vi "LogSpectra.vi"(7 "Area":i32, 8 "error in (no error)":errorcluster, 9 "50mA Spectra":cluster{"Wavelength":dbl[], "EL Spectrum":dbl[]}, 10 "20mA Spectra":cluster{"Wavelength":dbl[], "EL Spectrum":dbl[]}, 11 "LotData in":refnum<class "LotData.lvclass">) -> (0 "error out":errorcluster, 2 "Boolean":bool=TRUE, 3 "LotData out":refnum<class "LotData.lvclass">)   [LabVIEW 2012, in "LotData.lvclass"]
uses:
  LotData.lvclass
  <vilib>/addons/database/NI_Database_API.lvlib
  <vilib>/addons/database/Connection.llb/DB Tools Open Connec (Path).vi
  <vilib>/addons/database/Auxilliary.llb/DB Tools Parameter Dir.ctl
  <vilib>/addons/database/Auxilliary.llb/DB Tools DataTypes.ctl
  <vilib>/addons/database/Auxilliary.llb/DB Tools Parameter Info.ctl
  <vilib>/addons/database/Command.llb/Cmd Set Parameter Value (C).vi
  <vilib>/addons/database/Command.llb/Cmd Delete.vi
  <vilib>/LVH/i3 JSON/i3-json.lvlib
  <vilib>/LVH/i3 JSON/JSON Generation/Create Value Files/Create Value - 1D Array Double.vi
  <vilib>/addons/database/Command.llb/Cmd Execute.vi
  <vilib>/addons/database/Recordset.llb/Rec Destroy - Command.vi
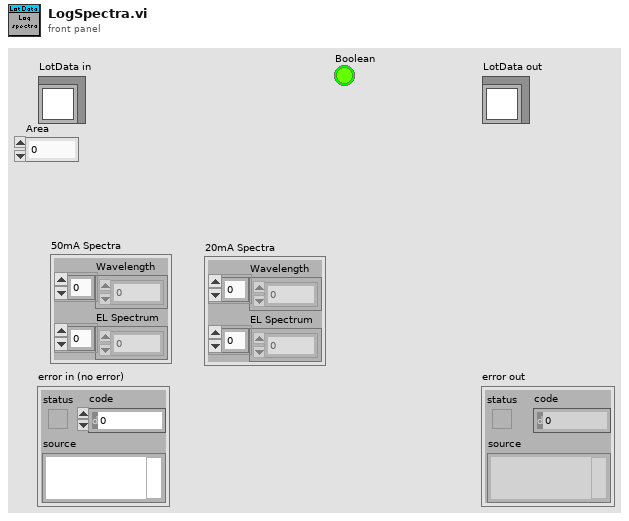
[diagram p1: front panel]
types:
  T1 = typedef "NI_Database_API.lvlib/DB Tools Parameter Info.ctl" = cluster{"parameter name":string, "type":T2, "direction":T3, "value":variant}
  T2 = typedef "NI_Database_API.lvlib/DB Tools DataTypes.ctl" = enum16{"String", "Long (I32)", "Single (SGL)", "Double (DBL)", "Date/Time", "Binary"}
  T3 = typedef "NI_Database_API.lvlib/DB Tools Parameter Dir.ctl" = enum32{"Input", "Output", "Input/Output", "Return Value"}
  T4 = typedef "MeasurementType.ctl" = enum16{"Initial", "Final"}
  T5 = typedef "NI_Database_API.lvlib/Conn ObjectReference.ctl" = refnum<k1>
  T6 = typedef "NI_Database_API.lvlib/Cmd ObjectReference.ctl" = refnum<k1>
  T7 = typedef "NI_Database_API.lvlib/Cmd-Rec Object Reference.ctl" = refnum<k1>
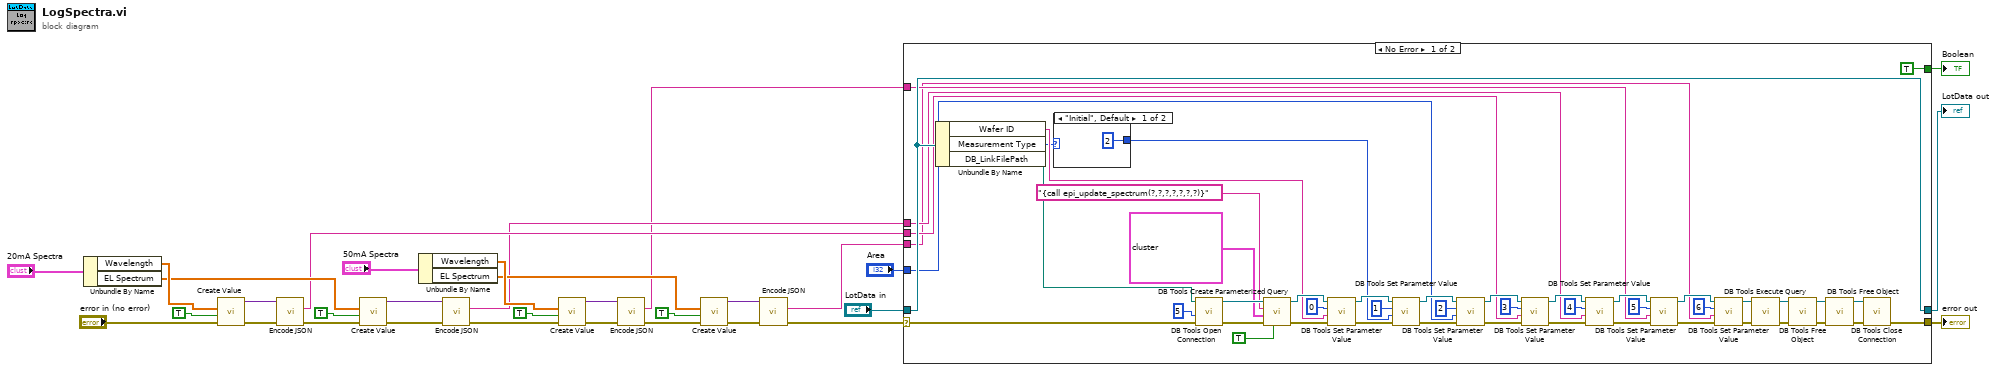
[diagram p0: block diagram]
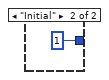
[diagram p2: hidden frame]
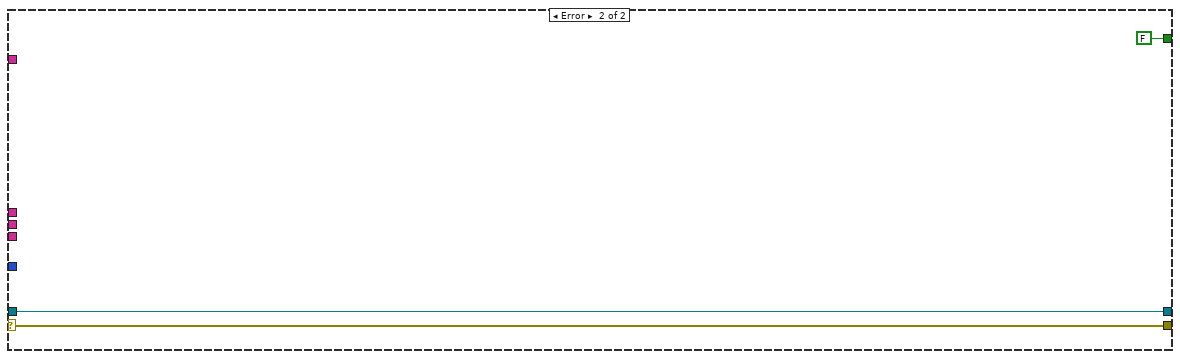
[diagram p3: hidden frame]
diagram:
  n1 = Unbundle By Name("20mA Spectra") -> ("Wavelength"=w27:dbl[], "EL Spectrum"=w21:dbl[])
  n2 = call-poly <vilib>:"Create Value.vi"("error in (no error)"="error in (no error)", "Create as 1D Array?"=TRUE, "1D Numeric"=w27) -> ("error out"=w18:errorcluster, "JSON Tree"=w17:variant)  [unwired: 7 in]
  n3 = call <vilib>:"Encode JSON.vi"("error in (no error)"=w18, "JSON Tree"=w17) -> ("error out"=w16:errorcluster, "String"=w14:string)  [unwired: 4 in]
  n4 = call-poly <vilib>:"Create Value.vi"("error in (no error)"=w16, "Create as 1D Array?"=TRUE, "1D Numeric"=w21) -> ("error out"=w6:errorcluster, "JSON Tree"=w7:variant)  [unwired: 7 in]
  n5 = Unbundle By Name("50mA Spectra") -> ("Wavelength"=w20:dbl[], "EL Spectrum"=w15:dbl[])
  n6 = call <vilib>:"Encode JSON.vi"("error in (no error)"=w6, "JSON Tree"=w7) -> ("error out"=w8:errorcluster, "String"=w5:string)  [unwired: 4 in]
  n7 = call-poly <vilib>:"Create Value.vi"("error in (no error)"=w8, "Create as 1D Array?"=TRUE, "1D Numeric"=w20) -> ("error out"=w12:errorcluster, "JSON Tree"=w13:variant)  [unwired: 7 in]
  n8 = call <vilib>:"Encode JSON.vi"("error in (no error)"=w12, "JSON Tree"=w13) -> ("error out"=w9:errorcluster, "String"=w4:string)  [unwired: 4 in]
  n9 = call-poly <vilib>:"Create Value.vi"("error in (no error)"=w9, "Create as 1D Array?"=TRUE, "1D Numeric"=w15) -> ("error out"=w10:errorcluster, "JSON Tree"=w11:variant)  [unwired: 7 in]
  n10 = call <vilib>:"Encode JSON.vi"("error in (no error)"=w10, "JSON Tree"=w11) -> ("error out"=w2:errorcluster, "String"=w3:string)  [unwired: 4 in]
  n11 = case shown="No Error" w2 {
    selector: w2 -> [w51 w85]
    tunnel: [w47 w85] -> w32
    tunnel: [w46 w84] -> w30
    tunnel: "LotData in" -> [w46 w84]
    tunnel: "Area" -> [w45 _]
    tunnel: w14 -> [w44 _]
    tunnel: w5 -> [w42 _]
    tunnel: w4 -> [w40 _]
    tunnel: w3 -> [w39 _]
    tunnel: [TRUE FALSE] -> w1
    frame No Error {
      n12 = Unbundle By Name(w46) -> ("Wafer ID"=w50:string, "Measurement Type"=w49:T4, "DB_LinkFilePath"=w34:path)
      n13 = case shown="Default, \"After\"" w49 {
        tunnel: [2 1] -> w48
        frame "Initial", Default {
        }
        frame "Initial" {
        }
      }
      n14 = call-poly <vilib>:"DB Tools Open Connection.vi"("error in (no error)"=w51, "connection timeout (15)"=5, "connection information"=w34) -> ("error out"=w78:errorcluster, "connection reference"=w79:T5)  [unwired: 5 in]
      n15 = call <vilib>:"DB Tools Create Parameterized Query.vi"("stored procedure? (F)"=TRUE, "error in (no error)"=w78, "parameters"=T1[] [{"parameter name"="wafer", "type"=enum."String", "direction"=enum."Input", "value"=variant}, {"parameter name"="test", "type"=enum."Single (SGL)", "direction"=enum."Input", "value"=variant}, {"parameter name"="area", "type"=enum."Single (SGL)", "direction"=enum."Input", "value"=variant}, {"parameter name"="wl", "type"=enum."String", "direction"=enum."Input", "value"=variant}, {"parameter name"="spect", "type"=enum."String", "direction"=enum."Input", "value"=variant}, {"parameter name"="wl50mA", "type"=enum."String", "direction"=enum."Input", "value"=variant}, {"parameter name"="spect50mA", "type"=enum."String", "direction"=enum."Input", "value"=variant}], "SQL query"="{call epi_update_spectrum(?,?,?,?,?,?,?)}", "connection reference"=w79) -> ("error out"=w75:errorcluster, "command reference"=w74:T6)  [unwired: 2 in, 1 out]
      n16 = call-poly <vilib>:"DB Tools Set Parameter Value.vi"("error in (no error)"=w75, "value"=w50, "parameter index"=0, "command reference"=w74) -> ("error out"=w52:errorcluster, "command reference out"=w62:T6)  [unwired: 4 in]
      n17 = call-poly <vilib>:"DB Tools Set Parameter Value.vi"("error in (no error)"=w52, "value"=w48, "parameter index"=1, "command reference"=w62) -> ("error out"=w53:errorcluster, "command reference out"=w61:T6)  [unwired: 4 in]
      n18 = call-poly <vilib>:"DB Tools Set Parameter Value.vi"("error in (no error)"=w53, "value"=w45, "parameter index"=2, "command reference"=w61) -> ("error out"=w54:errorcluster, "command reference out"=w60:T6)  [unwired: 4 in]
      n19 = call-poly <vilib>:"DB Tools Set Parameter Value.vi"("error in (no error)"=w54, "value"=w44, "parameter index"=3, "command reference"=w60) -> ("error out"=w55:errorcluster, "command reference out"=w43:T6)  [unwired: 4 in]
      n20 = call-poly <vilib>:"DB Tools Set Parameter Value.vi"("error in (no error)"=w55, "value"=w42, "parameter index"=4, "command reference"=w43) -> ("error out"=w56:errorcluster, "command reference out"=w59:T6)  [unwired: 4 in]
      n21 = call-poly <vilib>:"DB Tools Set Parameter Value.vi"("error in (no error)"=w56, "value"=w40, "parameter index"=5, "command reference"=w59) -> ("error out"=w57:errorcluster, "command reference out"=w58:T6)  [unwired: 4 in]
      n22 = call-poly <vilib>:"DB Tools Set Parameter Value.vi"("error in (no error)"=w57, "value"=w39, "parameter index"=6, "command reference"=w58) -> ("error out"=w38:errorcluster, "command reference out"=w37:T6)  [unwired: 4 in]
      n23 = call-poly <vilib>:"DB Tools Execute Query.vi"("error in (no error)"=w38, "command reference"=w37) -> ("error out"=w71:errorcluster, "command-recordset reference"=w72:T7)  [unwired: 6 in]
      n24 = call-poly <vilib>:"DB Tools Free Object.vi"("error in (no error)"=w71, "command-recordset reference"=w72) -> ("error out"=w73:errorcluster, "command reference"=w70:T6)  [unwired: 8 in]
      n25 = call-poly <vilib>:"DB Tools Free Object.vi"("error in (no error)"=w73, "command reference"=w70) -> ("error out"=w68:errorcluster, "connection reference"=w69:T5)  [unwired: 8 in]
      n26 = call <vilib>:"DB Tools Close Connection.vi"("error in (no error)"=w68, "connection reference"=w69) -> ("error out"=w47:errorcluster)  [unwired: 5 in]
    }
    frame Error {
    }
  }
  "error out" <- w32
  "LotData out" <- w30
  "Boolean" <- w1
